vi "Abort Stream.vi"(8 "error in (no error)":errorcluster, 11 "File Response in":refnum<class "File Response.lvclass">) -> (0 "error out":errorcluster, 3 "File Response out":refnum<class "File Response.lvclass">)   [LabVIEW 2020, in "HTTP Utils.lvlib" / "File Response.lvclass"]
uses:
  File Response.lvclass
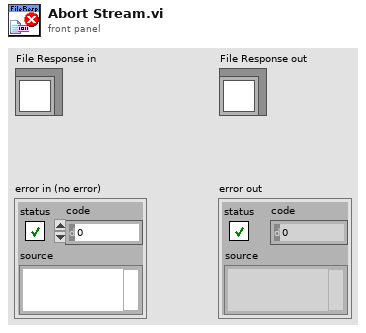
[diagram p1: front panel]
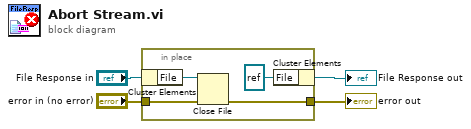
[diagram p0: block diagram]
diagram:
  n1 = in-place {
    in-place-border: "error in (no error)" -> [w6]
    in-place-border: [w5] -> w2
    n2 = in-place-cluster #1("File Response in") -> ("File"=w7:refnum<file>)
    n3 = Close File(refnum=w7, error in=w6) -> (error out=w5:errorcluster)  [unwired: 1 out]
    n4 = in-place-cluster #1("File"=refnum<file> refnum) -> (→"File Response out":refnum<class "File Response.lvclass">)
  }
  "error out" <- w2
